vi "json Insert I32 - array path.vi"(8 "error in (no error)":errorcluster, 9 "anything":i32, 10 "path":string[](array[string]), 11 "JSON Document in":refnum<class "JSON Document.lvclass">) -> (0 "error out":errorcluster, 1 "replaced?":bool, 3 "JSON Document out":refnum<class "JSON Document.lvclass">)   [LabVIEW 2015, in "JSON Document.lvclass"]
uses:
  JSON Document.lvclass
  json Insert I32 - string path.vi
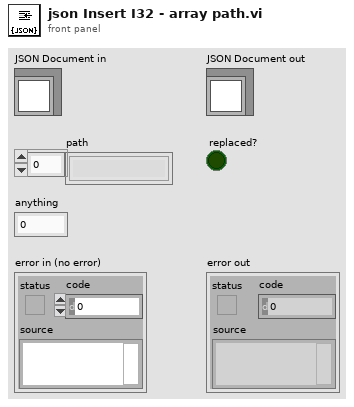
[diagram p1: front panel]
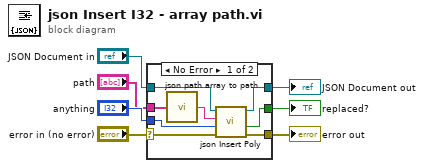
[diagram p0: block diagram]
diagram:
  n1 = case shown="No Error" "error in (no error)" {
    selector: "error in (no error)" -> [w11 w17]
    tunnel: [w10 w17] -> w6
    tunnel: [w9 w16] -> w4
    tunnel: "JSON Document in" -> [w14 w16]
    tunnel: "anything" -> [w12 _]
    tunnel: "path" -> [w13 _]
    tunnel: [w8 _] -> w1
    frame No Error {
      n2 = call "json path array to path.vi"("path"=w13) -> ("String"=w15:string)
      n3 = call-poly "json Insert Poly.vi"("error in (no error)"=w11, "anything"=w12, "path"=w15, "JSON Document in"=w14) -> ("error out"=w10:errorcluster, "replaced?"=w8:bool, "JSON Document out"=w9:refnum<class "JSON Document.lvclass">)  [unwired: 5 in]
    }
    frame Error {
    }
  }
  "error out" <- w6
  "JSON Document out" <- w4
  "replaced?" <- w1
